vi "RampFunction.vi"(10 "Max Rate per Iteration":dbl, 11 "Input":dbl(slide) scale=-1.0..1.0) -> (3 "Output":dbl(slide) scale=-1.0..1.0)   [LabVIEW 2016]
panel:
  out "Waveform Chart":T1(graph)
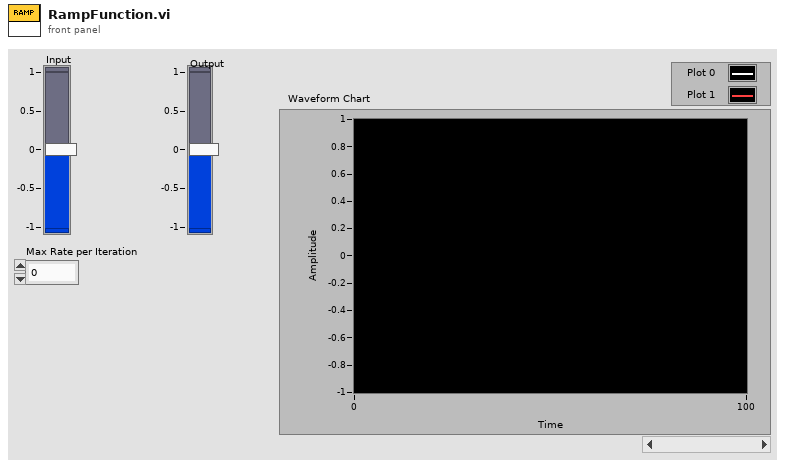
[diagram p1: front panel]
types:
  T1 = cluster{"Joystick Input":dbl, "Joystick Input":dbl}
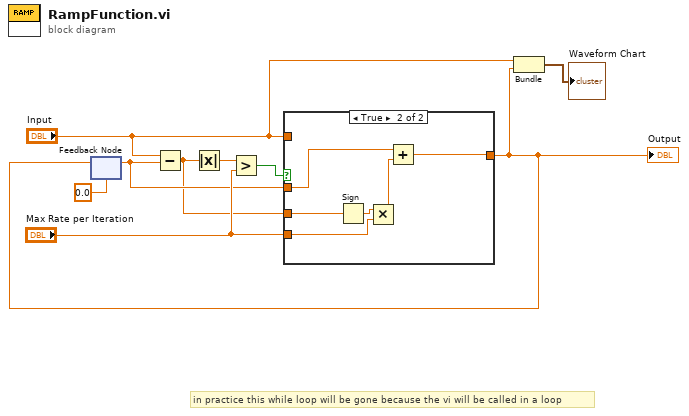
[diagram p0: block diagram]
diagram:
  # "in practice this while loop will be gone because the vi will be called in a loop"
  n1 = feedback #1(0.0) -> (w4:dbl)
  n2 = Subtract(x="Input", y=w4) -> (x-y=w1:dbl)
  n3 = Absolute Value(x=w1) -> (abs(x)=w6:dbl)
  n4 = Greater?(x=w6, y="Max Rate per Iteration") -> (0:w8:bool)
  n5 = case shown="True" w8 {
    tunnel: "Max Rate per Iteration" -> [_ w14]
    tunnel: "Input" -> [w10 _]
    tunnel: [w10 w16] -> w3
    tunnel: w4 -> [_ w12]
    tunnel: w1 -> [_ w11]
    frame False {
    }
    frame True {
      n6 = Sign(1:w11) -> (0:w15:dbl)
      n7 = Multiply(x=w15, y=w14) -> (x*y=w13:dbl)
      n8 = Add(x=w12, y=w13) -> (x+y=w16:dbl)
    }
  }
  "Output" <- w3
  n9 = feedback-in #1(w3) -> ()
  n10 = Bundle("Input"="Input", "Input"=w3) -> (→"Waveform Chart":cluster{"Input":dbl, "Input":dbl})  [unwired: 1 in]
